vi "rotate 2D array V2.vi"() -> ()   [LabVIEW 2010]
panel:
  out "x":i32
  out "y":i32
  out "yr":i32
  out "x r":i32
  out "element":cdb
  out "array in 2":cdb[][](array[numeric])
  out "output array":cdb[][](array[numeric])
  out "array out":cdb[][](array[numeric])
  in  "rotate y":i32
  in  "rotate x":i32
  in  "array in":cdb[][](array[numeric])=[[0.0+0.0i, 1.0+0.0i, 2.0+0.0i, 3.0+0.0i], [4.0+0.0i, 0.0+0.0i, 0.0+0.0i, 0.0+0.0i], [7.0+0.0i, 0.0+0.0i, 11.0+0.0i, 0.0+0.0i], [99.0+0.0i, 0.0+0.0i, 0.0+0.0i, 0.0+0.0i]]
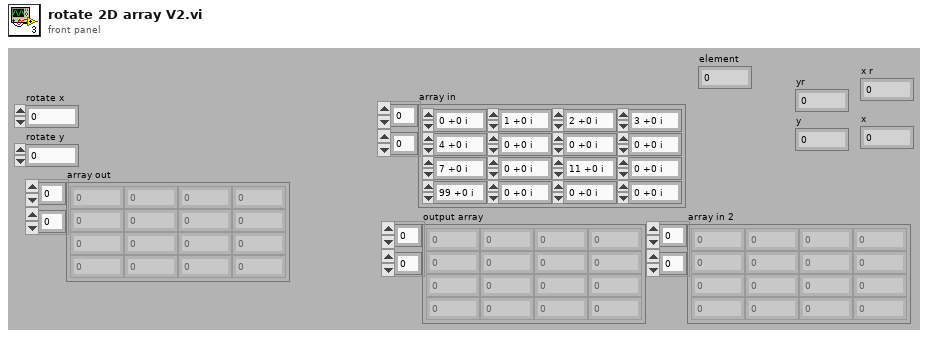
[diagram p1: front panel]
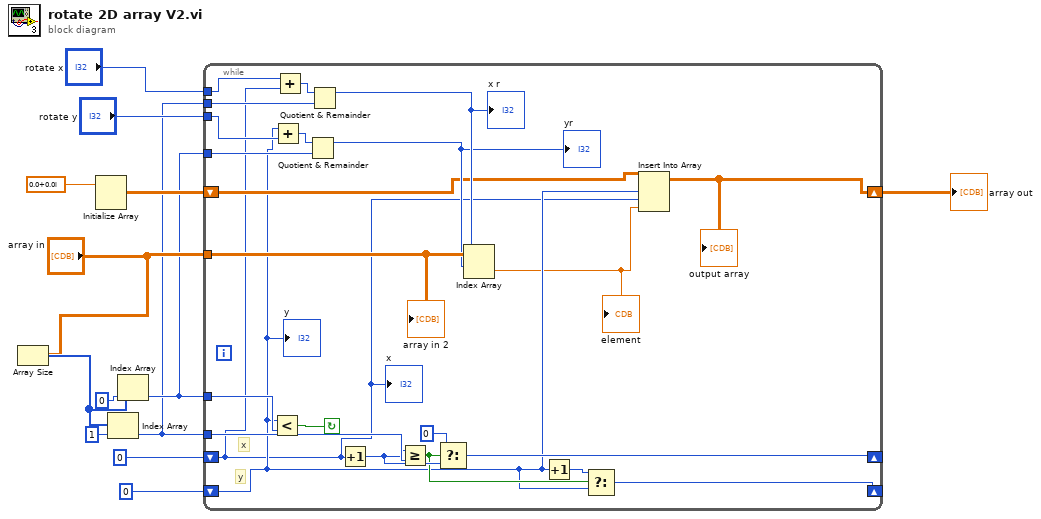
[diagram p0: block diagram]
diagram:
  n1 = Array Size(array="array in") -> (size(s)=w10:i32[])
  n2 = Initialize Array(cdb 0.0+0.0i ("element")) -> (w9:cdb[][])  [unwired: 2 in]
  n3 = Index Array(array=w10, index=1) -> (element=w1:i32)
  n4 = Index Array(array=w10, index=0) -> (element=w2:i32)
  n5 = while {
    shift-right: [w17] -> w5
    shift-left: w9 -> [w18]
    tunnel: "rotate y" -> [w34]
    tunnel: "array in" -> [w28]
    tunnel: "rotate x" -> [w26]
    shift-right: [w29] -> _
    shift-left: 0 -> [w15]
    shift-right: [w20] -> _
    shift-left: 0 -> [w16]
    tunnel: w2 -> [w33]
    tunnel: w1 -> [w32]
    tunnel: w2 -> [w23]
    tunnel: w1 -> [w22]
    stop <- w36 continue-if-true
    # "y"
    # "x"
    n6 = Less?(x=w16, y=w33) -> (x < y?=w36:bool)
    n7 = Add(x=w16, y=w34) -> (x+y=w35:i32)
    n8 = Add(x=w26, y=w15) -> (x+y=w27:i32)
    n9 = Quotient & Remainder(x=w35, y=w23) -> (x-y*floor(x/y)=w24:i32)  [unwired: 1 out]
    "yr" <- w24
    n10 = Quotient & Remainder(x=w27, y=w22) -> (x-y*floor(x/y)=w25:i32)  [unwired: 1 out]
    "x r" <- w25
    n11 = Increment(x=w15) -> (x+1=w30:i32)
    n12 = Greater Or Equal?(x=w30, y=w32) -> (x >= y?=w21:bool)
    n13 = Select(t=0, s=w21, f=w30) -> (s? t:f=w29:i32)
    n14 = Index Array(array=w28, index (row)=w24, index (col)=w25) -> (element=w14:cdb)
    "element" <- w14
    n15 = Increment(x=w16) -> (x+1=w19:i32)
    n16 = Select(t=w19, s=w21, f=w16) -> (s? t:f=w20:i32)
    n17 = Insert Into Array(array=w18, index (row)=w16, index (col)=w15, new element=w14) -> (w17:cdb[][])
    "output array" <- w17
    "array in 2" <- w28
    "y" <- w16
    "x" <- w15
  }
  "array out" <- w5
